vi "SaveCalibrationsToFile.vi"   [LabVIEW 2016]
uses:
  Configurations.vi
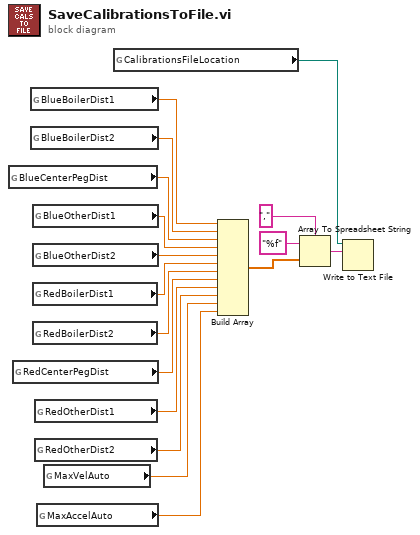
[diagram p0: block diagram]
diagram:
  n1 = global read "Configurations.vi" "BlueCenterPegDist"() -> (w15:dbl)
  n2 = global read "Configurations.vi" "RedCenterPegDist"() -> (w10:dbl)
  n3 = global read "Configurations.vi" "BlueBoilerDist1"() -> (w17:dbl)
  n4 = global read "Configurations.vi" "BlueBoilerDist2"() -> (w16:dbl)
  n5 = global read "Configurations.vi" "BlueOtherDist1"() -> (w14:dbl)
  n6 = global read "Configurations.vi" "BlueOtherDist2"() -> (w13:dbl)
  n7 = global read "Configurations.vi" "RedBoilerDist1"() -> (w12:dbl)
  n8 = global read "Configurations.vi" "RedBoilerDist2"() -> (w11:dbl)
  n9 = global read "Configurations.vi" "RedOtherDist1"() -> (w9:dbl)
  n10 = global read "Configurations.vi" "RedOtherDist2"() -> (w8:dbl)
  n11 = global read "Configurations.vi" "MaxAccelAuto"() -> (w1:dbl)
  n12 = global read "Configurations.vi" "MaxVelAuto"() -> (w2:dbl)
  n13 = global read "Configurations.vi" "CalibrationsFileLocation"() -> (w3:path)
  n14 = Build Array(w17, w16, w15, w14, w13, w12, w11, w10, w9, w8, w2, w1) -> (w7:dbl[])
  n15 = Array To Spreadsheet String(delimiter (Tab)=",", array=w7, 3:"%f" ("format string")) -> (spreadsheet string=w4:string)
  n16 = Write to Text File(file (use dialog)=w3, text=w4) -> ()  [unwired: 2 in, 3 out]
